vi "Measure.vi"(11 "WT1600 in":refnum<class "WT1600.lvclass">) -> (1 "Read Strings":string, 2 "Measure":dbl[](array[numeric]) format="%^.4e", 3 "WT1600 in 2":refnum<class "WT1600.lvclass">)   [LabVIEW 2012, in "Universal Power Meter.lvlib" / "WT1600.lvlib" / "WT1600.lvclass"]
uses:
  WT1600.lvclass
  WT1600.lvclass/WT1600.ctl
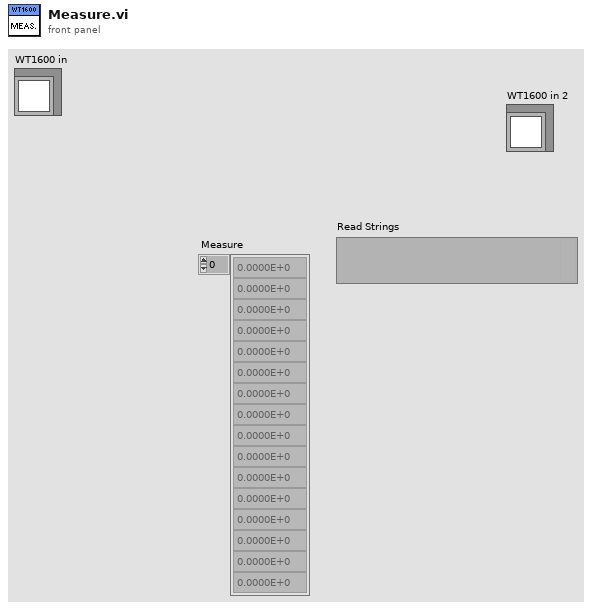
[diagram p1: front panel]
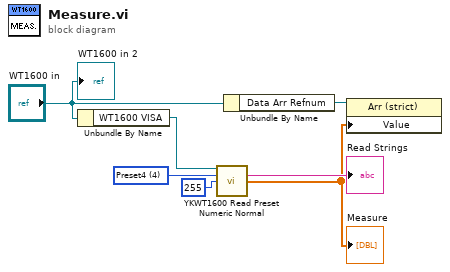
[diagram p0: block diagram]
diagram:
  w7 = u16 4 items=["", "Preset1", "Preset2", "Preset3", "Preset4"] ("Preset (2: Preset 2)")
  n1 = Unbundle By Name("WT1600 in") -> ("WT1600 VISA"=w1:refnum<visa-resource-name>)
  n2 = call <instrlib>:"YKWT1600 Read Preset Numeric Normal.vi"("VISA session"=w1, "Preset (2: Preset 2)"=w7, "Number of Item (15)"=u16 255) -> ("Read Strings"=→"Read Strings":string, "Measure"=w2:dbl[])  [unwired: 9 in, 2 out]
  "Measure" <- w2
  n3 = Unbundle By Name("WT1600 in") -> ("Data Arr Refnum"=w3:refnum<vi>)
  n4 = property class="Arr (strict)"(reference=w3, "Value"=w2) -> ()  [unwired: 1 in, 2 out]
  "WT1600 in 2" <- "WT1600 in"
